vi "工况电流加载.vi"(4 "Bool引用句柄":refnum<vi>, 7 "数值":i32, 8 "error in (no error)":errorcluster, 9 "电源台数":dbl, 10 "数组":dbl[][](array[numeric]), 11 "VISA resource name out":refnum<visa-resource-name>) -> (0 "error out":errorcluster, 3 "VISA resource name out 2":refnum<visa-resource-name>, 6 "已完成循环":i32)   [LabVIEW 2021]
uses:
  <instrlib>/TDK-Lambda G Series/TDK-Lambda G Series.lvlib
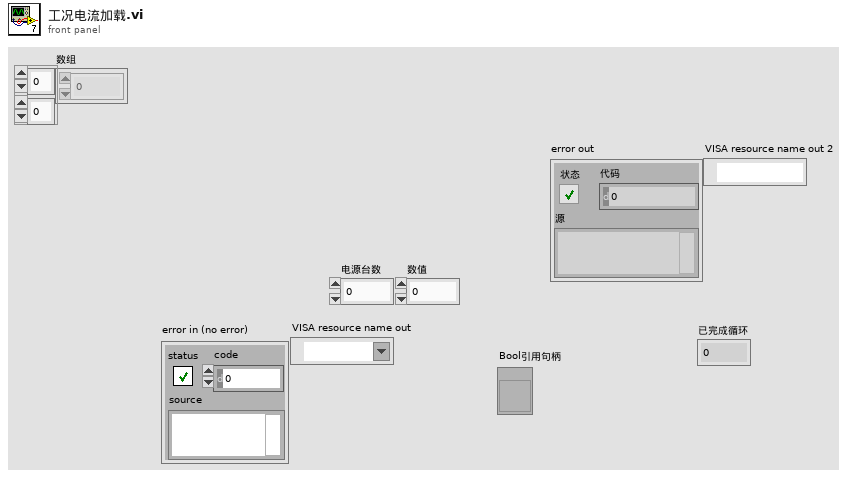
[diagram p1: front panel]
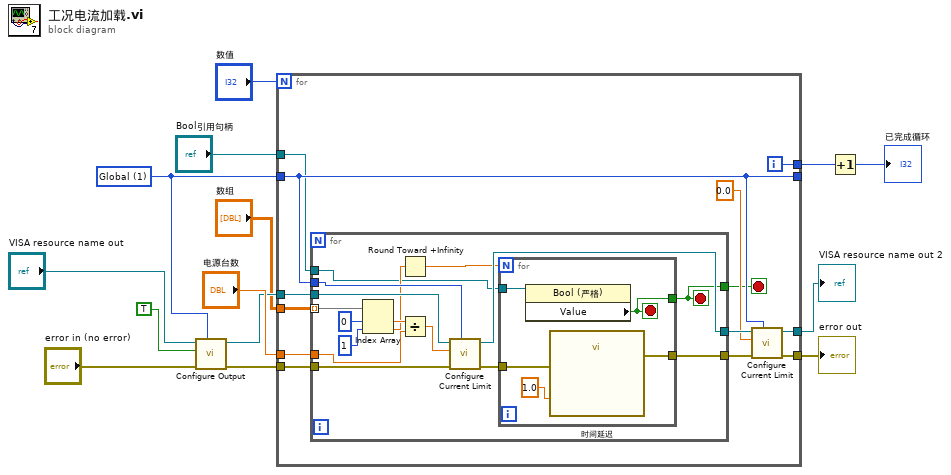
[diagram p0: block diagram]
diagram:
  w9 = u16 1 items=["Single", "Global"] ("Globalize (0: Single)")
  n1 = call <instrlib>:"Configure Output.vi"("Globalize (0: Single)"=w9, "error in (no error)"="error in (no error)", "Enable Output (False)"=TRUE, "VISA resource name"="VISA resource name out") -> ("error out"=w12:errorcluster, "VISA resource name out"=w7:refnum<visa-resource-name>)  [unwired: 6 in]
  n2 = for {
    N: "数值" -> [_]
    tunnel: "数组" -> [w20]
    tunnel: w9 -> [w19]
    tunnel: [w19] -> _
    tunnel: "电源台数" -> [w18]
    tunnel: w12 -> [w23]
    tunnel: [w22] -> w4
    tunnel: w7 -> [w25]
    tunnel: [w21] -> w3
    tunnel: "Bool引用句柄" -> [w16]
    tunnel: [w15] -> w14
    i -> [w15]
    stop <- w17 stop-if-true
    n3 = for {
      tunnel: w20 -> [w43] mode=indexing
      tunnel: w25 -> [w40]
      tunnel: w23 -> [w39]
      tunnel: [w37] -> w27
      tunnel: [w36] -> w26
      tunnel: w19 -> [w35]
      tunnel: w18 -> [w32]
      tunnel: [w28] -> w17
      tunnel: w16 -> [w29]
      stop <- w28 stop-if-true
      n4 = Index Array(array=w43, index #1=0 ("索引"), index #2=1 ("索引")) -> (element #1=w34:dbl, element #2=w31:dbl)
      n5 = Round Toward +Infinity(x=w31) -> (ceil(x): smallest int >= x=w30:dbl)
      n6 = Divide(x=w34, y=w32) -> (x/y=w33:dbl)
      n7 = call <instrlib>:"Configure Current Limit.vi"("Globalize (0: Single)"=w35, "error in (no error)"=w39, "Current Limit (0A)"=w33, "VISA resource name"=w40) -> ("error out"=w38:errorcluster, "VISA resource name out"=w36:refnum<visa-resource-name>)  [unwired: 6 in]
      n8 = for {
        N: w30 -> [_]
        tunnel: w38 -> [w48]
        tunnel: [w47] -> w37
        tunnel: w29 -> [w45]
        tunnel: [w44] -> w28
        stop <- w44 stop-if-true
        n9 = property class="Bool (严格)"(reference=w45) -> ("Value"=w44:bool)  [unwired: 1 in, 2 out]
        n10 = call "时间延迟"("error in (no error)"=w48, "Delay Time (s)"=1.0) -> ("error out"=w47:errorcluster)  [unwired: 9 in]
      }
    }
    n11 = call <instrlib>:"Configure Current Limit.vi"("Globalize (0: Single)"=w19, "error in (no error)"=w27, "Current Limit (0A)"=0.0, "VISA resource name"=w26) -> ("error out"=w22:errorcluster, "VISA resource name out"=w21:refnum<visa-resource-name>)  [unwired: 6 in]
  }
  "error out" <- w4
  "VISA resource name out 2" <- w3
  n12 = Increment(x=w14) -> (x+1=→"已完成循环":i32)
